vi "Flush Buffer.vi"(8 "error in":errorcluster, 11 "Buffer in":refnum<data-value>) -> (0 "error out":errorcluster, 2 "elements":variant[](array[variant]), 3 "Buffer":refnum<data-value>)   [LabVIEW 2013, in "VariantBuffer.lvclass"]
doc: "This VI returns data from the ring buffer starting from the oldest data and ending with the newest.\n\nThe data is duplicated at the output so this VI allocates new place in the memory for the output."
uses:
  VariantBuffer.lvclass
  VariantBuffer.lvclass/VariantBuffer.ctl
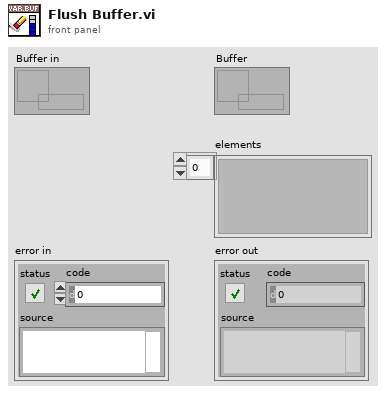
[diagram p1: front panel]
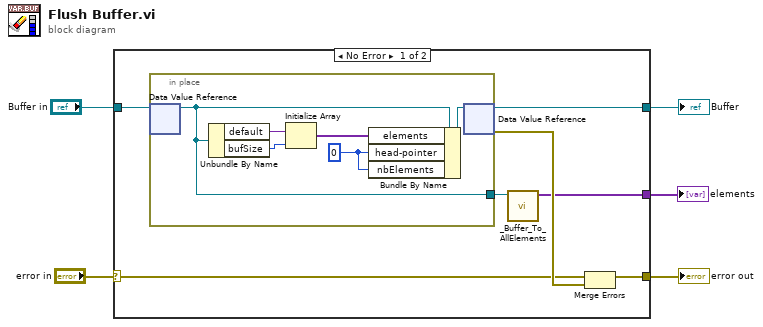
[diagram p0: block diagram]
diagram:
  n1 = case shown="No Error" "error in" {
    selector: "error in" -> [w8 w19]
    tunnel: "Buffer in" -> [w9 w20]
    tunnel: [w12 w20] -> w4
    tunnel: [w11 w19] -> w1
    tunnel: [w6 _] -> w3
    frame No Error {
      n2 = in-place {
        in-place-border: [w13] -> w7
        w17 = 0 ("Index")
        n3 = in-place-dvr #1(w9) -> (w13:refnum<class "VariantBuffer.lvclass">)  [unwired: 1 out]
        n4 = Unbundle By Name(w13) -> ("default"=w14:variant, "bufSize"=w16:i32)
        n5 = Initialize Array(w14, w16) -> (w18:variant[])
        n6 = Bundle By Name(cluster=w13, "elements"=w18, "head-pointer"=w17, "nbElements"=w17) -> (w15:refnum<class "VariantBuffer.lvclass">)
        n7 = in-place-dvr #1(w15) -> (w12:refnum<data-value>, w10:errorcluster)
      }
      n8 = call "_Buffer_To_AllElements.vi"("Buffer"=w7) -> ("elements"=w6:variant[])  [unwired: 10 in]
      n9 = Merge Errors(w8, w10) -> (w11:errorcluster)
    }
    frame Error {
    }
  }
  "error out" <- w1
  "Buffer" <- w4
  "elements" <- w3
